vi "HMI Labview PWM motor DERECK.vi"() -> ()   [LabVIEW 2025]
uses:
  <vilib>/MakerHub/LINX/LMH-LINX.lvlib
  <vilib>/MakerHub/LINX/Public/Utilities/Open Serial.vi
  <vilib>/MakerHub/LINX/Public/Peripherals/PWM/PWM Set Duty Cycle 1 Chan.vi
panel:
  in  "PDW %":dbl(slide) scale=0.0..10.0
  in  "Serial Port":refnum<visa-resource-name>="N/A"
  in  "stop":bool
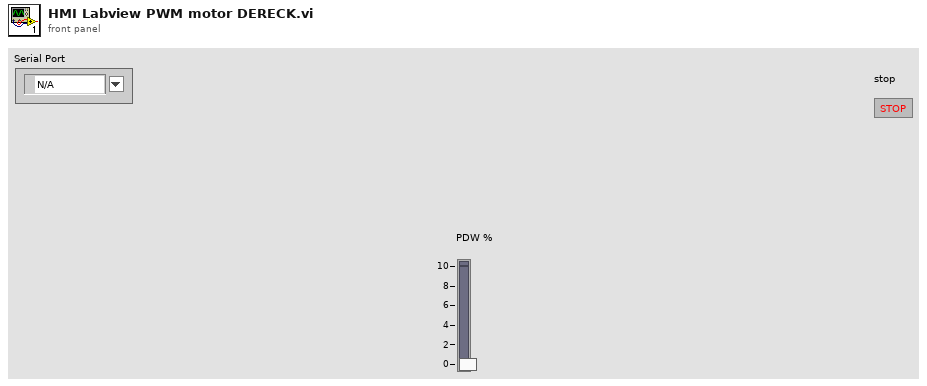
[diagram p1: front panel]
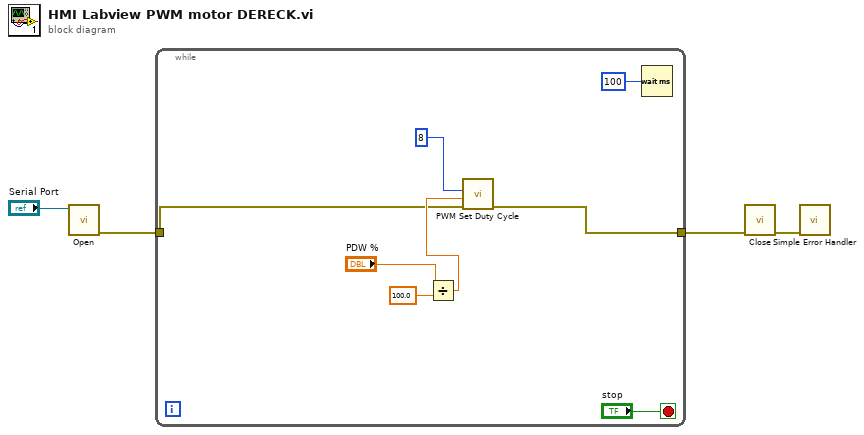
[diagram p0: block diagram]
diagram:
  n1 = call-poly <vilib>:"Open.vi"("Serial Port"="Serial Port") -> ("Error Out"=w3:errorcluster)  [unwired: 8 in, 2 out]
  n2 = while {
    tunnel: w3 -> [w9]
    tunnel: [w8] -> w2
    stop <- "stop" stop-if-true
    n3 = Divide(x="PDW %", y=100.0) -> (x/y=w10:dbl)
    n4 = call-poly <vilib>:"PWM Set Duty Cycle.vi"("Error In"=w9, "Duty Cycle (0-1)"=w10, "PWM Channel"=u8 8) -> ("Error Out"=w8:errorcluster)  [unwired: 7 in, 1 out]
    n5 = Wait (ms)(milliseconds to wait=u32 100) -> ()  [unwired: 1 out]
  }
  n6 = call <vilib>:"Close.vi"("Error In"=w2) -> ("Error Out"=w4:errorcluster)  [unwired: 10 in]
  n7 = call <vilib>:"Simple Error Handler.vi"("error in (no error)"=w4) -> ()  [unwired: 4 in, 5 out]
